vi "CMI Sync V3 Set Source.vi"(8 "error in":errorcluster, 9 "HV range (1kV)":T1=enum."1kV", 10 "Source (Internal)":T2, 11 "session in":T3={"VISA"="", "baud rate [bd/s]"=115200, "source"=enum."Auto", "hv range"=enum."1kV", "fsrc is fixed"=FALSE, "fsrc [Hz]"=10000000.0, "freq integ [s]"=1.0, "freq filter"=5, "trig level"=enum."TTL 5V", "chn1 mode"=enum."Source divider", "chn1 level"=enum."Positive 5V", "chn2 mode"=enum."Source divider", "chn2 level"=enum."Positive 5V", "chn2 div"=1, "chn3 mode"=enum."Chn 1 Active", "chn3 level"=enum."Positive 5V", "chn1 div entry"=enum."Calculate nearest divisor from measured fx", "chn1 dev limit [%]"=1.0, "chn1 check dev"=FALSE} {"chn2 div" min=1 max=100000000 step=1; "fsrc [Hz]" format="%_8p"}) -> (0 "error out":errorcluster, 3 "session out":T3={"VISA"="", "baud rate [bd/s]"=115200, "source"=enum."Auto", "hv range"=enum."1kV", "fsrc is fixed"=FALSE, "fsrc [Hz]"=10000000.0, "freq integ [s]"=1.0, "freq filter"=5, "trig level"=enum."TTL 5V", "chn1 mode"=enum."Source divider", "chn1 level"=enum."Positive 5V", "chn2 mode"=enum."Source divider", "chn2 level"=enum."Positive 5V", "chn2 div"=1, "chn3 mode"=enum."Chn 1 Active", "chn3 level"=enum."Positive 5V", "chn1 div entry"=enum."Calculate nearest divisor from measured fx", "chn1 dev limit [%]"=1.0, "chn1 check dev"=FALSE} {"chn2 div" min=1 max=100000000 step=1; "fsrc [Hz]" format="%_8p"})   [LabVIEW 2020, in "AWG.lvlib" / "CMI Sync Unit V3.lvlib"]
doc: "Sets reference clock source. For HV input it also sets HV range."
uses:
  CMI Sync Unit V3.lvlib
  CMI Sync V3 session.ctl
  CMI Sync V3 Reference Clock Source.ctl
  CMI Sync V3 HV input Range.ctl
  CMI Sync V3 Trigger Input Level.ctl
  CMI Sync V3 Channel 1 Mode.ctl
  CMI Sync V3 Channel Output Levels.ctl
  CMI Sync V3 Channel 2 Mode.ctl
  CMI Sync V3 Channel 3 Mode.ctl
  CMI Sync V3 Channel 1 Divisor Entry Mode.ctl
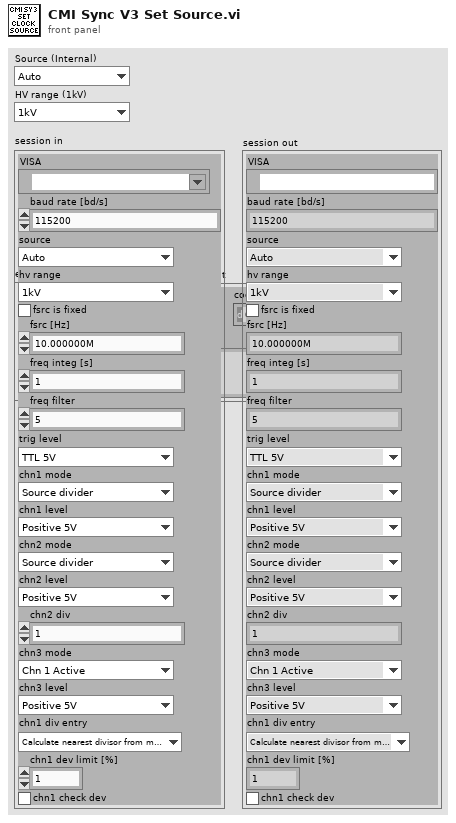
[diagram p1: front panel]
types:
  T1 = typedef "AWG.lvlib/CMI Sync Unit V3.lvlib/CMI Sync V3 HV input Range.ctl" = enum16{"10V", "60V", "250V", "1kV"}
  T2 = typedef "AWG.lvlib/CMI Sync Unit V3.lvlib/CMI Sync V3 Reference Clock Source.ctl" = enum16{"Auto", "Internal", "Logic", "Sine", "HV"}
  T3 = typedef "AWG.lvlib/CMI Sync Unit V3.lvlib/CMI Sync V3 session.ctl" = cluster{"VISA":refnum<visa-resource-name>, "baud rate [bd/s]":i32, "source":T2, "hv range":T1, "fsrc is fixed":bool, "fsrc [Hz]":dbl, "freq integ [s]":dbl, "freq filter":i32, "trig level":T4, "chn1 mode":T5, "chn1 level":T6, "chn2 mode":T7, "chn2 level":T6, "chn2 div":i32, "chn3 mode":T8, "chn3 level":T6, "chn1 div entry":T9, "chn1 dev limit [%]":dbl, "chn1 check dev":bool}
  T4 = typedef "AWG.lvlib/CMI Sync Unit V3.lvlib/CMI Sync V3 Trigger Input Level.ctl" = enum16{"LVCMOS 3V3", "TTL 5V"}
  T5 = typedef "AWG.lvlib/CMI Sync Unit V3.lvlib/CMI Sync V3 Channel 1 Mode.ctl" = enum16{"Source divider", "DDS absolute", "DDS ratio", "DDS ratio M/N"}
  T6 = typedef "AWG.lvlib/CMI Sync Unit V3.lvlib/CMI Sync V3 Channel Output Levels.ctl" = enum16{"Positive 3V3", "Negative 3V3", "Positive 5V", "Negative 5V"}
  T7 = typedef "AWG.lvlib/CMI Sync Unit V3.lvlib/CMI Sync V3 Channel 2 Mode.ctl" = enum16{"Source divider", "Chn 1 divide"}
  T8 = typedef "AWG.lvlib/CMI Sync Unit V3.lvlib/CMI Sync V3 Channel 3 Mode.ctl" = enum16{"Chn 1 Active", "Chn 2 Active", "Chn 1 Trigger", "Chn 2 Trigger", "Gate", "PPS", "10MHz"}
  T9 = typedef "AWG.lvlib/CMI Sync Unit V3.lvlib/CMI Sync V3 Channel 1 Divisor Entry Mode.ctl" = enum16{"Set divisor directly", "Calculate nearest divisor from measured fx"}
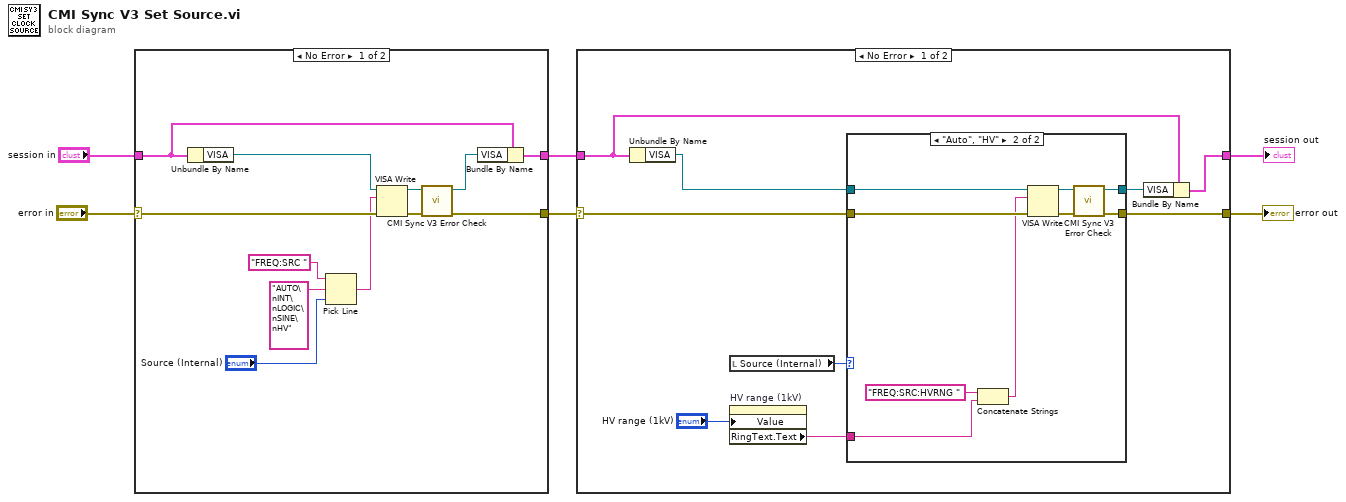
[diagram p0: block diagram]
diagram:
  n1 = case shown="No Error" "error in" {
    selector: "error in" -> [w16 w20]
    tunnel: "session in" -> [w18 w19]
    tunnel: [w17 w19] -> w3
    tunnel: [w8 w20] -> w4
    frame No Error {
      n2 = Unbundle By Name(w18) -> ("VISA"=w15:refnum<visa-resource-name>)
      n3 = Pick Line(string ("")="FREQ:SRC ", multi-line string="AUTO\nINT\nLOGIC\nSINE\nHV", line index="Source (Internal)") -> (output string=w12:string)
      n4 = VISA Write(VISA resource name=w15, write buffer=w12, error in (no error)=w16) -> (VISA resource name out=w9:refnum<visa-resource-name>, error out=w10:errorcluster)  [unwired: 1 out]
      n5 = call "CMI Sync V3 Error Check.vi"("error in"=w10, "VISA in"=w9) -> ("error out"=w8:errorcluster, "VISA out"=w7:refnum<visa-resource-name>)  [unwired: 7 in, 1 out]
      n6 = Bundle By Name(cluster=w18, "VISA"=w7) -> (w17:T3)
    }
    frame Error {
    }
  }
  n7 = case shown="No Error" w4 {
    selector: w4 -> [w23 w42]
    tunnel: w3 -> [w29 w41]
    tunnel: [w28 w41] -> w1
    tunnel: [w22 w42] -> w2
    frame No Error {
      n8 = Unbundle By Name(w29) -> ("VISA"=w24:refnum<visa-resource-name>)
      n9 = local read "Source (Internal)"() -> (w25:T2)
      n10 = property on="HV range (1kV)" class="Enum (strict)"("Value"="HV range (1kV)") -> ("RingText.Text"=w26:string)  [unwired: 2 in, 2 out]
      n11 = case shown="\"Auto\", \"HV\"" w25 {
        tunnel: w23 -> [w31 w40]
        tunnel: w26 -> [_ w37]
        tunnel: [w31 w32] -> w22
        tunnel: w24 -> [w30 w36]
        tunnel: [w30 w33] -> w21
        frame Default {
        }
        frame "Auto", "HV" {
          n12 = Concatenate Strings("FREQ:SRC:HVRNG " ("string"), w37) -> (w38:string)
          n13 = VISA Write(VISA resource name=w36, write buffer=w38, error in (no error)=w40) -> (VISA resource name out=w34:refnum<visa-resource-name>, error out=w35:errorcluster)  [unwired: 1 out]
          n14 = call "CMI Sync V3 Error Check.vi"("error in"=w35, "VISA in"=w34) -> ("error out"=w32:errorcluster, "VISA out"=w33:refnum<visa-resource-name>)  [unwired: 7 in, 1 out]
        }
      }
      n15 = Bundle By Name(cluster=w29, "VISA"=w21) -> (w28:T3)
    }
    frame Error {
    }
  }
  "error out" <- w2
  "session out" <- w1
